vi "Angle_Dist.vi"(1 "TargetAngle":dbl, 2 "CurrentAngle":dbl) -> (0 "Distance":dbl)   [LabVIEW 2017]
panel:
  # "Inputs"
  # "Output"
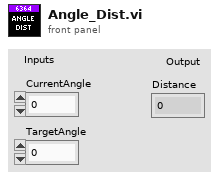
[diagram p1: front panel]
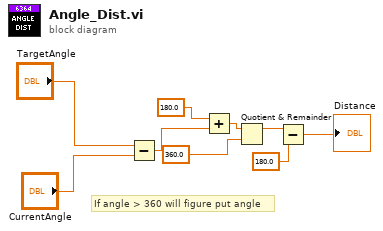
[diagram p0: block diagram]
diagram:
  # "If angle > 360 will figure put angle"
  n1 = Subtract(x="TargetAngle", y="CurrentAngle") -> (x-y=w6:dbl)
  n2 = Add(x=180.0, y=w6) -> (x+y=w5:dbl)
  n3 = Quotient & Remainder(x=w5, y=360.0) -> (x-y*floor(x/y)=w3:dbl)  [unwired: 1 out]
  n4 = Subtract(x=w3, y=180.0) -> (x-y=→"Distance":dbl)
